vi "SubVI_AutoDrive_Auto.vi"(8 "error in (no error)":errorcluster) -> (0 "error out":errorcluster, 1 "EncoderLeft(Inches)":i32=14, 2 "EncoderRight(Inches)":i32=14)   [LabVIEW 2017]
uses:
  <vilib>/Rock Robotics/WPI/ThirdParty/Phoenix-LabVIEW/Motor Controller/Controls/CTRE_Phoenix_MotorControl_ControlMode.ctl
  <vilib>/Rock Robotics/WPI/ThirdParty/Phoenix-LabVIEW/Motor Controller/Controls/CTRE_Phoenix_MotorControl_FeedbackDevice.ctl
  <vilib>/Rock Robotics/WPI/ThirdParty/Phoenix-LabVIEW/Motor Controller/Get/CTRE_Phoenix_MotorController_GetSelectedSensorData.vi
panel:
  in  "LeftDriveValue":dbl=40000.0
  in  "RightDriveValue":dbl=40000.0
  in  "F 2":dbl=0.2
  in  "D 2":dbl=0.1
  in  "I 2":dbl
  in  "P 2":dbl=0.1
  in  "F":dbl=0.2
  in  "D":dbl=0.1
  in  "I":dbl
  in  "P":dbl=0.1
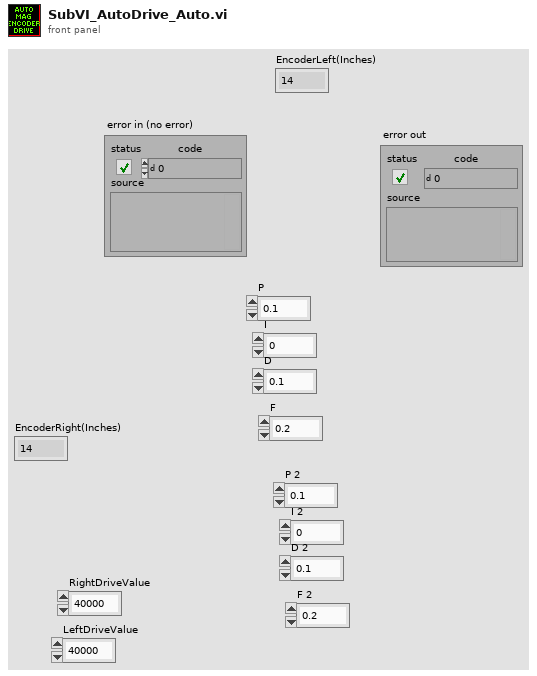
[diagram p1: front panel]
types:
  T1 = typedef "CTRE_Phoenix_MotorControl_FeedbackDevice.ctl" = i8
  T2 = typedef "CTRE_Phoenix_MotorControl_ControlMode.ctl" = u16
  T3 = typedef "WPI_MotorControlDeviceRef.ctl" = cluster{"DeviceStatus":errorcluster, "Type":T4, "PWM":cluster{"PWM Channel":T5, "DeadBand":T6}, "CAN":cluster{"Device Number":u8, "SetOutput VI Ref":variant, "GetOutput VI Ref":variant, "Enable VI Ref":variant, "Disable VI Ref":variant, "Data":variant}, "Invert":bool, "DIO PWM":cluster{"PWM \"Enable\" Channel":T5, "DIOChannel":T7, "PWM Rate":dbl}}
  T4 = typedef "WPI_MotorControlType.ctl" = enum16{"PWM", "CAN", "DIO PWM"}
  T5 = typedef "FPGA_DIOPWMChannel.ctl" = enum8{"PWM 0", "PWM 1", "PWM 2", "PWM 3", "PWM 4", "PWM 5", "PWM 6", "PWM 7", "PWM 8", "PWM 9", "PWM MXP 0", "PWM MXP 1", "PWM MXP 2", "PWM MXP 3", "PWM MXP 4", "PWM MXP 5", "PWM MXP 6", "PWM MXP 7", "PWM MXP 8", "PWM MXP 9", "Invalid"}
  T6 = typedef "WPI_PWMDeadband.ctl" = cluster{"Name":string, "maxPositivePwm":i32, "minPositivePwm":i32, "centerPwm":i32, "maxNegativePwm":i32, "minNegativePwm":i32, "angularRange":u16}
  T7 = typedef "FPGA_DIOChannel.ctl" = enum8{"DIO 0", "DIO 1", "DIO 2", "DIO 3", "DIO 4", "DIO 5", "DIO 6", "DIO 7", "DIO 8", "DIO 9", "DIO MXP 0", "DIO MXP 1", "DIO MXP 2", "DIO MXP 3", "DIO MXP 4", "DIO MXP 5", "DIO MXP 6", "DIO MXP 7", "DIO MXP 8", "DIO MXP 9", "DIO MXP 10", "DIO MXP 11", "DIO MXP 12", "DIO MXP 13", "DIO MXP 14", "DIO MXP 15", "SPI Port CS1", "SPI Port CS2", "SPI Port CS3", "SPI Port MISO", "SPI Port MOSI", "Invalid"}
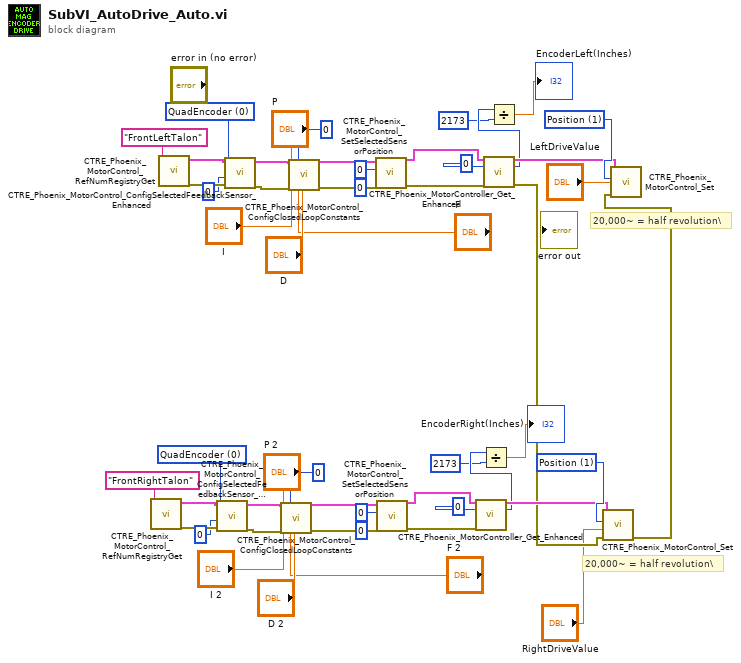
[diagram p0: block diagram]
diagram:
  w28 = T1 0 items=["None"=-1, "QuadEncoder"=0, "Analog"=2, "Tachometer"=4, "Pulse Width Encoded Position"=8, "Sensor Sum (S0 + S1)"=9, "Sensor Difference (D0 - D1)"=10, "Remote Source 0"=11, "Remote Source 1"=12, "Software Emulated"=15] ("Feedback Device")
  w34 = T2 1 items=["PercentOutput"=0, "Position"=1, "Velocity"=2, "Current"=3, "Follower"=5, "MotionProfile"=6, "MotionMagic"=7, "MotionMagicArc"=8, "MotionProfileArc"=10, "Disabled"=15] ("Control Mode")
  w46 = T1 0 items=["None"=-1, "QuadEncoder"=0, "Analog"=2, "Tachometer"=4, "Pulse Width Encoded Position"=8, "Sensor Sum (S0 + S1)"=9, "Sensor Difference (D0 - D1)"=10, "Remote Source 0"=11, "Remote Source 1"=12, "Software Emulated"=15] ("Feedback Device")
  w52 = T2 1 items=["PercentOutput"=0, "Position"=1, "Velocity"=2, "Current"=3, "Follower"=5, "MotionProfile"=6, "MotionMagic"=7, "MotionMagicArc"=8, "MotionProfileArc"=10, "Disabled"=15] ("Control Mode")
  # "20,000~ = half revolution\\"
  # "20,000~ = half revolution\\"
  n1 = call <vilib>:"CTRE_Phoenix_MotorControl_RefNumRegistryGet.vi"("refnum name"="FrontRightTalon") -> ("error out"=w29:errorcluster, "PhoenixMotorControlDevRef"=w30:T3)  [unwired: 9 in]
  n2 = call <vilib>:"CTRE_Phoenix_MotorControl_RefNumRegistryGet.vi"("refnum name"="FrontLeftTalon") -> ("error out"=w47:errorcluster, "PhoenixMotorControlDevRef"=w48:T3)  [unwired: 9 in]
  n3 = call <vilib>:"CTRE_Phoenix_MotorControl_ConfigSelectedFeedbackSensor_Enhanced.vi"("error in (no error)"=w29, "pidLoopIdx"=0, "Feedback Device"=w28, "PhoenixMotorControlDevRef"=w30) -> ("error out"=w25:errorcluster, "PhoenixMotorControlDevRef"=w26:T3)  [unwired: 6 in]
  n4 = call <vilib>:"CTRE_Phoenix_MotorControl_ConfigSelectedFeedbackSensor_Enhanced.vi"("error in (no error)"=w47, "pidLoopIdx"=0, "Feedback Device"=w46, "PhoenixMotorControlDevRef"=w48) -> ("error out"=w43:errorcluster, "PhoenixMotorControlDevRef"=w44:T3)  [unwired: 6 in]
  n5 = call <vilib>:"CTRE_Phoenix_MotorControl_ConfigClosedLoopConstants.vi"("PhoenixMotorControlDevRef"=w26, "slotIdx"=0, "P"="P 2", "I"="I 2", "D"="D 2", "error in (no error)"=w25, "F"="F 2") -> ("PhoenixMotorControlDevRef"=w15:T3, "error out"=w14:errorcluster)  [unwired: 7 in]
  n6 = call <vilib>:"CTRE_Phoenix_MotorControl_ConfigClosedLoopConstants.vi"("PhoenixMotorControlDevRef"=w44, "slotIdx"=0, "P"="P", "I"="I", "D"="D", "error in (no error)"=w43, "F"="F") -> ("PhoenixMotorControlDevRef"=w10:T3, "error out"=w9:errorcluster)  [unwired: 7 in]
  n7 = call <vilib>:"CTRE_Phoenix_MotorControl_SetSelectedSensorPosition.vi"("error in (no error)"=w9, "pidLoopIdx"=u32 0, "New Sensor Position"=0, "PhoenixMotorControlDevRef"=w10) -> ("error out"=w8:errorcluster, "PhoenixMotorControlDevRef"=w11:T3)  [unwired: 6 in]
  n8 = call <vilib>:"CTRE_Phoenix_MotorControl_SetSelectedSensorPosition.vi"("error in (no error)"=w14, "pidLoopIdx"=u32 0, "New Sensor Position"=0, "PhoenixMotorControlDevRef"=w15) -> ("error out"=w13:errorcluster, "PhoenixMotorControlDevRef"=w16:T3)  [unwired: 6 in]
  n9 = call-poly <vilib>:"CTRE_Phoenix_MotorController_Get_Enhanced.vi"("PhoenixMotorControlDevRef"=w16, "pidLoopIdx"=u32 0, "error in"=w13) -> ("PhoenixMotorControlDevRef"=w32:T3, "Position (Raw Sensor Units)"=w20:i32)  [unwired: 9 in, 2 out]
  n10 = Divide(x=w20, y=2173) -> (x/y=→"EncoderRight(Inches)":dbl)
  n11 = call-poly <vilib>:"CTRE_Phoenix_MotorController_Get_Enhanced.vi"("PhoenixMotorControlDevRef"=w11, "pidLoopIdx"=u32 0, "error in"=w8) -> ("PhoenixMotorControlDevRef"=w50:T3, "Position (Raw Sensor Units)"=w38:i32, "error out"=w4:errorcluster)  [unwired: 9 in, 1 out]
  n12 = Divide(x=w38, y=2173) -> (x/y=→"EncoderLeft(Inches)":dbl)
  n13 = call <vilib>:"CTRE_Phoenix_MotorControl_Set.vi"("error in (no error)"=w4, "Output"="RightDriveValue", "Control Mode"=w34, "PhoenixMotorControlDevRef"=w32) -> ("error out"=w3:errorcluster)  [unwired: 6 in, 1 out]
  n14 = call <vilib>:"CTRE_Phoenix_MotorControl_Set.vi"("error in (no error)"=w3, "Output"="LeftDriveValue", "Control Mode"=w52, "PhoenixMotorControlDevRef"=w50) -> ()  [unwired: 6 in, 2 out]
